vi "BRig_RT_comm_tcp_write_RTwrite__RunState_Trial_selResult__v2.vi"(7 "input_dataTrial":u16[][](array[numeric]), 10 "iReward_or_iError":bool, 11 "input_dataCurrent":u16[](array[numeric])) -> (2 "output_strCmd":string)   [LabVIEW 2014]
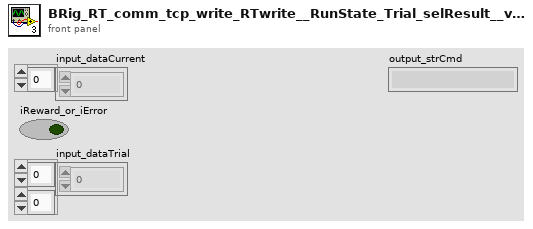
[diagram p1: front panel]
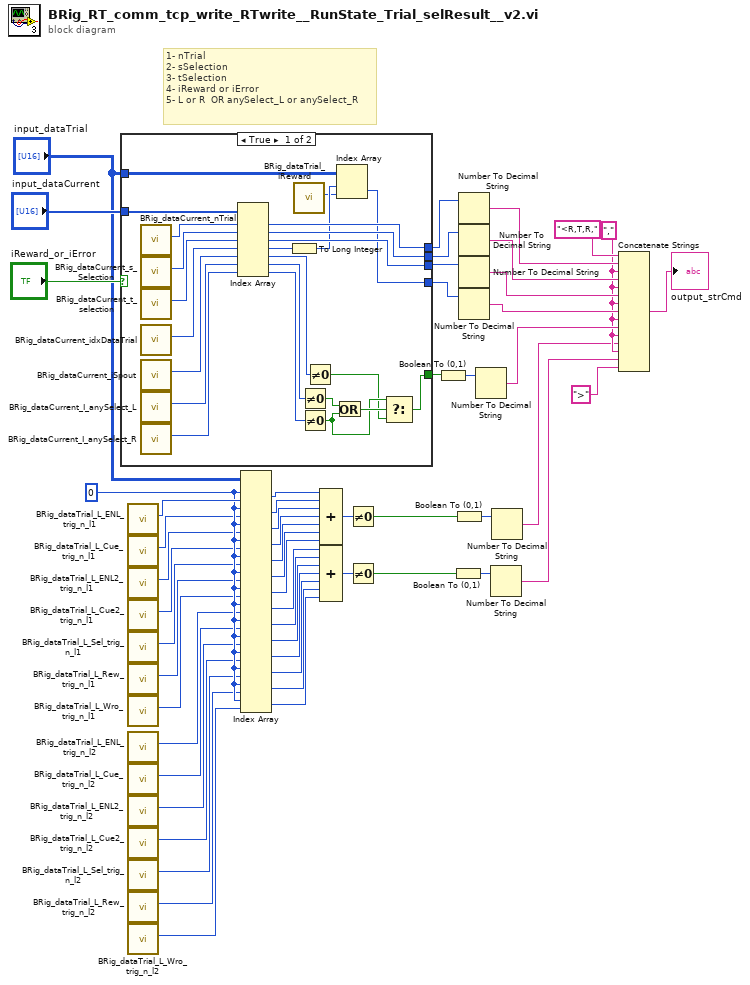
[diagram p0: block diagram]
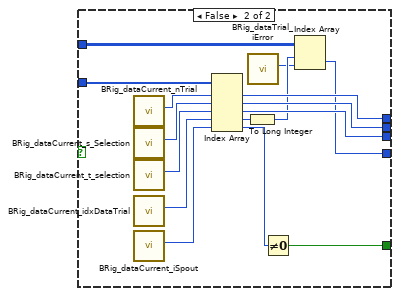
[diagram p2: hidden frame]
diagram:
  w28 = 0
  w33 = "," ("string")
  # "1- nTrial\n2- sSelection\n3- tSelection\n4- iReward or iError\n5- L or R  OR anySelect_L or anySelect_R"
  n1 = case shown="True" "iReward_or_iError" {
    tunnel: "input_dataCurrent" -> [w78 w94]
    tunnel: [w75 w91] -> w50
    tunnel: [w74 w90] -> w49
    tunnel: [w73 w89] -> w48
    tunnel: "input_dataTrial" -> [w69 w85]
    tunnel: [w67 w84] -> w47
    tunnel: [w56 w81] -> w52
    frame True {
      n2 = call "BRig_dataCurrent_nTrial.vi"() -> ("output_nTrial"=w79:i32)  [unwired: 11 in]
      n3 = call "BRig_dataCurrent_s_Selection.vi"() -> ("output_s_Selection"=w77:i32)  [unwired: 11 in]
      n4 = call "BRig_dataCurrent_t_selection.vi"() -> ("output_t_selection"=w76:i32)  [unwired: 11 in]
      n5 = call "BRig_dataCurrent_idxDataTrial.vi"() -> ("output_idxDataTrial"=w72:i32)  [unwired: 11 in]
      n6 = call "BRig_dataCurrent_iSpout.vi"() -> ("output_iSpout"=w66:i32)  [unwired: 11 in]
      n7 = call "BRig_dataCurrent_I_anySelect_L.vi"() -> ("output_IanySelect_L"=w65:i32)  [unwired: 11 in]
      n8 = call "BRig_dataCurrent_I_anySelect_R.vi"() -> ("output_IanySelect_R"=w64:i32)  [unwired: 11 in]
      n9 = Index Array(array=w78, index #1=w79, index #2=w77, index #3=w76, index #4=w72, index #5=w66, index #6=w65, index #7=w64) -> (element #1=w75:u16, element #2=w74:u16, element #3=w73:u16, element #4=w71:u16, element #5=w58:u16, element #6=w63:u16, element #7=w62:u16)
      n10 = To Long Integer(number=w71) -> (32bit integer=w70:i32)
      n11 = call "BRig_dataTrial_iReward.vi"() -> ("output_iReward"=w68:i32)  [unwired: 11 in]
      n12 = Not Equal To 0?(x=w63) -> (x != 0?=w61:bool)
      n13 = Not Equal To 0?(x=w62) -> (x != 0?=w59:bool)
      n14 = Not Equal To 0?(x=w58) -> (x != 0?=w57:bool)
      n15 = Or(x=w61, y=w59) -> (x .or. y?=w60:bool)
      n16 = Index Array(array=w69, index (row)=w70, index (col)=w68) -> (element=w67:u16)
      n17 = Select(t=w59, s=w60, f=w57) -> (s? t:f=w56:bool)
    }
    frame False {
      n18 = call "BRig_dataCurrent_nTrial.vi"() -> ("output_nTrial"=w95:i32)  [unwired: 11 in]
      n19 = call "BRig_dataCurrent_s_Selection.vi"() -> ("output_s_Selection"=w93:i32)  [unwired: 11 in]
      n20 = call "BRig_dataCurrent_t_selection.vi"() -> ("output_t_selection"=w92:i32)  [unwired: 11 in]
      n21 = call "BRig_dataCurrent_idxDataTrial.vi"() -> ("output_idxDataTrial"=w88:i32)  [unwired: 11 in]
      n22 = call "BRig_dataCurrent_iSpout.vi"() -> ("output_iSpout"=w83:i32)  [unwired: 11 in]
      n23 = Index Array(array=w94, index #1=w95, index #2=w93, index #3=w92, index #4=w88, index #5=w83) -> (element #1=w91:u16, element #2=w90:u16, element #3=w89:u16, element #4=w87:u16, element #5=w82:u16)
      n24 = To Long Integer(number=w87) -> (32bit integer=w86:i32)
      n25 = call "BRig_dataTrial_iError.vi"() -> ("output_iError"=w80:i32)  [unwired: 11 in]
      n26 = Not Equal To 0?(x=w82) -> (x != 0?=w81:bool)
      n27 = Index Array(array=w85, index (row)=w86, index (col)=w80) -> (element=w84:u16)
    }
  }
  n28 = call "BRig_dataTrial_L_ENL_trig_n_l1.vi"() -> ("output_L_ENL_trig_n_l1"=w29:i32)  [unwired: 11 in]
  n29 = call "BRig_dataTrial_L_Cue_trig_n_l1.vi"() -> ("output_L_Cue_trig_n_l1"=w27:i32)  [unwired: 11 in]
  n30 = call "BRig_dataTrial_L_ENL2_trig_n_l1.vi"() -> ("output_L_ENL2_trig_n_l1"=w26:i32)  [unwired: 11 in]
  n31 = call "BRig_dataTrial_L_Cue2_trig_n_l1.vi"() -> ("output_L_Cue2_trig_n_l1"=w25:i32)  [unwired: 11 in]
  n32 = call "BRig_dataTrial_L_Sel_trig_n_l1.vi"() -> ("output_L_Sel_trig_n_l1"=w24:i32)  [unwired: 11 in]
  n33 = call "BRig_dataTrial_L_Rew_trig_n_l1.vi"() -> ("output_L_Reward_trig_n_l1"=w4:i32)  [unwired: 11 in]
  n34 = call "BRig_dataTrial_L_Wro_trig_n_l1.vi"() -> ("output_L_Wrong_trig_n_l1"=w2:i32)  [unwired: 11 in]
  n35 = call "BRig_dataTrial_L_ENL_trig_n_l2.vi"() -> ("output_L_ENL_trig_n_l2"=w23:i32)  [unwired: 11 in]
  n36 = call "BRig_dataTrial_L_Cue_trig_n_l2.vi"() -> ("output_L_Cue_trig_n_l2"=w22:i32)  [unwired: 11 in]
  n37 = call "BRig_dataTrial_L_ENL2_trig_n_l2.vi"() -> ("output_L_ENL2_trig_n_l2"=w21:i32)  [unwired: 11 in]
  n38 = call "BRig_dataTrial_L_Cue2_trig_n_l2.vi"() -> ("output_L_Cue2_trig_n_l2"=w20:i32)  [unwired: 11 in]
  n39 = call "BRig_dataTrial_L_Sel_trig_n_l2.vi"() -> ("output_L_Sel_trig_n_l2"=w19:i32)  [unwired: 11 in]
  n40 = call "BRig_dataTrial_L_Rew_trig_n_l2.vi"() -> ("output_L_Reward_trig_n_l2"=w3:i32)  [unwired: 11 in]
  n41 = call "BRig_dataTrial_L_Wro_trig_n_l2.vi"() -> ("output_L_Wrong_trig_n_l2"=w1:i32)  [unwired: 11 in]
  n42 = Index Array(array="input_dataTrial", index (row) #1=w28, index (col) #1=w29, index (row) #2=w28, index (col) #2=w27, index (row) #3=w28, index (col) #3=w26, index (row) #4=w28, index (col) #4=w25, index (row) #5=w28, index (col) #5=w24, index (row) #6=w28, index (col) #6=w4, index (row) #7=w28, index (col) #7=w2, index (row) #8=w28, index (col) #8=w23, index (row) #9=w28, index (col) #9=w22, index (row) #10=w28, index (col) #10=w21, index (row) #11=w28, index (col) #11=w20, index (row) #12=w28, index (col) #12=w19, index (row) #13=w28, index (col) #13=w3, index (row) #14=w28, index (col) #14=w1) -> (element #1=w18:u16, element #2=w17:u16, element #3=w16:u16, element #4=w15:u16, element #5=w14:u16, element #6=w13:u16, element #7=w12:u16, element #8=w11:u16, element #9=w10:u16, element #10=w9:u16, element #11=w8:u16, element #12=w7:u16, element #13=w6:u16, element #14=w5:u16)
  n43 = Compound Arithmetic op=ADD(w18, w17, w16, w15, w14, w13, w12) -> (w40:u16)
  n44 = Compound Arithmetic op=ADD(w11, w10, w9, w8, w7, w6, w5) -> (w39:u16)
  n45 = Not Equal To 0?(x=w40) -> (x != 0?=w36:bool)
  n46 = Not Equal To 0?(x=w39) -> (x != 0?=w35:bool)
  n47 = Boolean To (0,1)(Boolean=w52) -> (0, 1=w51:i16)
  n48 = Boolean To (0,1)(Boolean=w35) -> (0, 1=w37:i16)
  n49 = Boolean To (0,1)(Boolean=w36) -> (0, 1=w38:i16)
  n50 = Number To Decimal String(number=w50) -> (decimal integer string=w46:string)  [unwired: 1 in]
  n51 = Number To Decimal String(number=w49) -> (decimal integer string=w45:string)  [unwired: 1 in]
  n52 = Number To Decimal String(number=w48) -> (decimal integer string=w44:string)  [unwired: 1 in]
  n53 = Number To Decimal String(number=w47) -> (decimal integer string=w43:string)  [unwired: 1 in]
  n54 = Number To Decimal String(number=w51) -> (decimal integer string=w42:string)  [unwired: 1 in]
  n55 = Number To Decimal String(number=w37) -> (decimal integer string=w31:string)  [unwired: 1 in]
  n56 = Number To Decimal String(number=w38) -> (decimal integer string=w32:string)  [unwired: 1 in]
  n57 = Concatenate Strings("<R,T,R," ("string"), w46, w33, w45, w33, w44, w33, w43, w33, w42, w33, w32, w33, w31, ">" ("string")) -> (→"output_strCmd":string)
